vi "S1500_S7Com_ISO_WRT(SubVI).vi"(4 "error in":errorcluster, 5 "timeout ms (25000)":i32, 6 "TPDU_In":T1 format="X%02x", 7 "connection ID in":refnum<k5>) -> (0 "error out":errorcluster, 3 "connection ID out":refnum<k5>)   [LabVIEW 2018]
doc: "Adds the ISO 8073 Header to the Protocol Data Unit (PDU) and calls the TPKT write subVI."
uses:
  S1500_test_S7Com_HexByteArray.ctl
  S1500_S7Com_HexByte.ctl
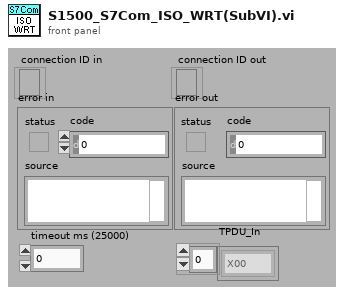
[diagram p1: front panel]
types:
  T1 = typedef "S1500_test_S7Com_HexByteArray.ctl" = T2[]
  T2 = typedef "S1500_S7Com_HexByte.ctl" = u8
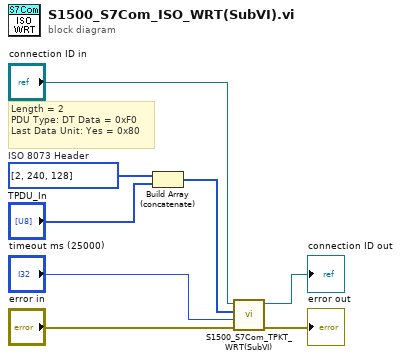
[diagram p0: block diagram]
diagram:
  w1 = u8[] [2, 240, 128]  # ISO 8073 Header
  # "Length = 2\nPDU Type: DT Data = 0xF0\nLast Data Unit: Yes = 0x80"
  n1 = Build Array (concatenate)(w1, "TPDU_In") -> (w3:T1)
  n2 = call "S1500_S7Com_TPKT_WRT(SubVI).vi"("error in"="error in", "timeout ms"="timeout ms (25000)", "TPDU_In"=w3, "connection ID in"="connection ID in") -> ("error out"=→"error out":errorcluster, "connection ID out"=→"connection ID out":refnum<k5>)  [unwired: 2 out]
